vi "4Linea1.vi"(11 "array":string[][](array[string])) -> (3 "x .or. y?":bool)   [LabVIEW 2020]
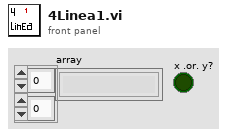
[diagram p1: front panel]
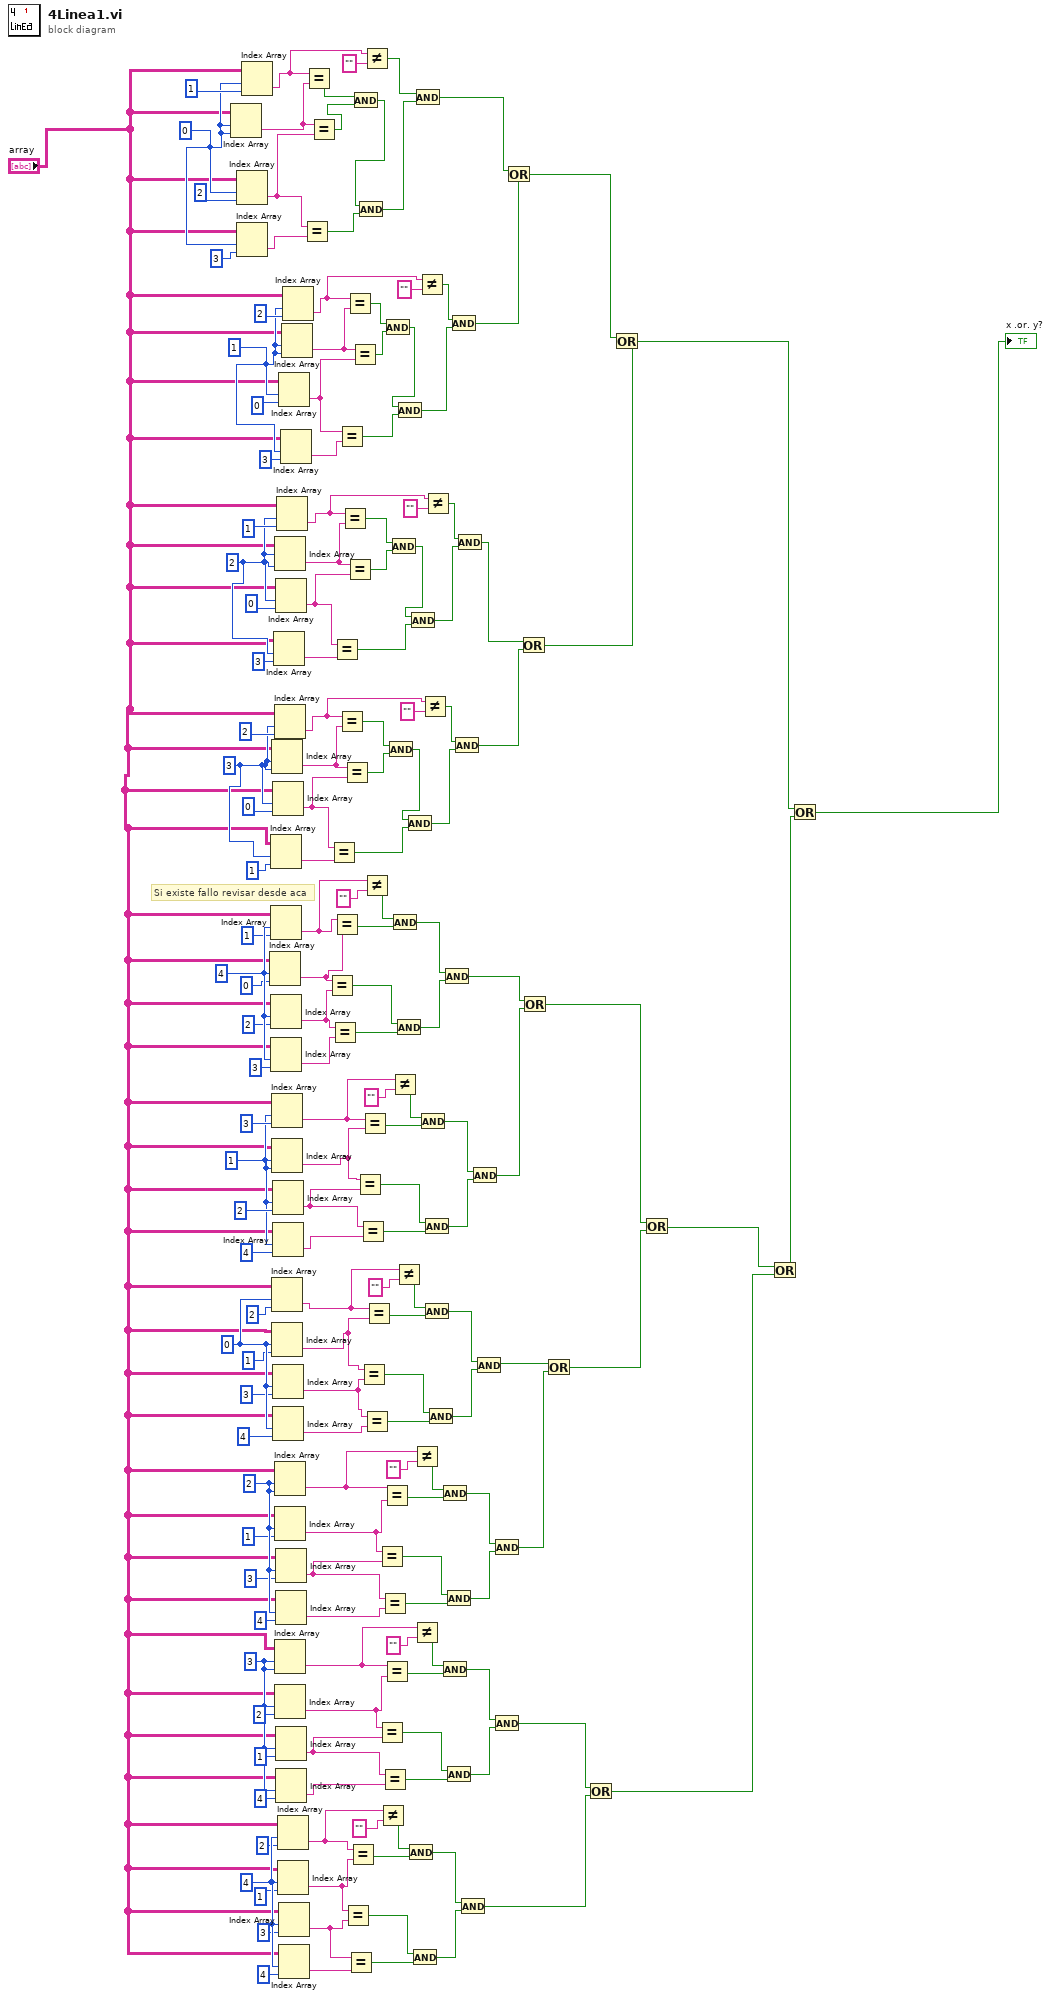
[diagram p0: block diagram]
diagram:
  w20 = 4 ("index (row)")
  w54 = 3 ("index (row)")
  w58 = 2 ("index (row)")
  w63 = 0 ("index (row)")
  w89 = 1 ("index (row)")
  w107 = 4 ("index (row)")
  w116 = 3
  w131 = 2
  w138 = 1
  w146 = 0
  # "Si existe fallo revisar desde aca"
  n1 = Index Array(array="array", index (row)=w146, index (col)=w146) -> (element=w171:string)
  n2 = Index Array(array="array", index (row)=w146, index (col)=2) -> (element=w144:string)
  n3 = Index Array(array="array", index (row)=w146, index (col)=3) -> (element=w143:string)
  n4 = Index Array(array="array", index (row)=w146, index (col)=1) -> (element=w152:string)
  n5 = Index Array(array="array", index (row)=w107, index (col)=0 ("disabled index (col)")) -> (element=w101:string)
  n6 = Index Array(array="array", index (row)=w116, index (col)=1) -> (element=w114:string)
  n7 = Index Array(array="array", index (row)=w107, index (col)=1 ("disabled index (col)")) -> (element=w102:string)
  n8 = Index Array(array="array", index (row)=w107, index (col)=2 ("disabled index (col)")) -> (element=w100:string)
  n9 = Index Array(array="array", index (row)=w107, index (col)=3 ("disabled index (col)")) -> (element=w99:string)
  n10 = Index Array(array="array", index (row)=w116, index (col)=w116) -> (element=w123:string)
  n11 = Index Array(array="array", index (row)=w89, index (col)=3 ("disabled index (col)")) -> (element=w80:string)
  n12 = Index Array(array="array", index (row)=w89, index (col)=w89) -> (element=w79:string)
  n13 = Index Array(array="array", index (row)=w63, index (col)=2 ("disabled index (col)")) -> (element=w69:string)
  n14 = Index Array(array="array", index (row)=w63, index (col)=1 ("disabled index (col)")) -> (element=w66:string)
  n15 = Index Array(array="array", index (row)=w116, index (col)=0) -> (element=w115:string)
  n16 = Index Array(array="array", index (row)=w89, index (col)=2 ("disabled index (col)")) -> (element=w78:string)
  n17 = Index Array(array="array", index (row)=w89, index (col)=4 ("disabled index (col)")) -> (element=w77:string)
  n18 = Index Array(array="array", index (row)=w63, index (col)=3 ("disabled index (col)")) -> (element=w68:string)
  n19 = Index Array(array="array", index (row)=w63, index (col)=4 ("disabled index (col)")) -> (element=w67:string)
  n20 = Index Array(array="array", index (row)=w131, index (col)=3) -> (element=w129:string)
  n21 = Index Array(array="array", index (row)=w131, index (col)=w131) -> (element=w165:string)
  n22 = Index Array(array="array", index (row)=w116, index (col)=2) -> (element=w119:string)
  n23 = Index Array(array="array", index (row)=w58, index (col)=w58) -> (element=w30:string)
  n24 = Index Array(array="array", index (row)=w58, index (col)=1 ("disabled index (col)")) -> (element=w29:string)
  n25 = Index Array(array="array", index (row)=w54, index (col)=w54) -> (element=w23:string)
  n26 = Index Array(array="array", index (row)=w54, index (col)=2) -> (element=w26:string)
  n27 = Index Array(array="array", index (row)=w131, index (col)=0) -> (element=w130:string)
  n28 = Index Array(array="array", index (row)=w58, index (col)=3 ("disabled index (col)")) -> (element=w28:string)
  n29 = Index Array(array="array", index (row)=w58, index (col)=4 ("disabled index (col)")) -> (element=w27:string)
  n30 = Index Array(array="array", index (row)=w54, index (col)=1) -> (element=w25:string)
  n31 = Index Array(array="array", index (row)=w54, index (col)=4) -> (element=w24:string)
  n32 = Index Array(array="array", index (row)=w131, index (col)=1) -> (element=w161:string)
  n33 = Index Array(array="array", index (row)=w20, index (col)=2) -> (element=w13:string)
  n34 = Index Array(array="array", index (row)=w20, index (col)=1) -> (element=w12:string)
  n35 = Index Array(array="array", index (row)=w138, index (col)=0) -> (element=w134:string)
  n36 = Index Array(array="array", index (row)=w20, index (col)=3) -> (element=w11:string)
  n37 = Index Array(array="array", index (row)=w20, index (col)=4) -> (element=w10:string)
  n38 = Index Array(array="array", index (row)=w138, index (col)=3) -> (element=w135:string)
  n39 = Index Array(array="array", index (row)=w138, index (col)=w138) -> (element=w168:string)
  n40 = Index Array(array="array", index (row)=w138, index (col)=2) -> (element=w155:string)
  n41 = Equal?(x=w144, y=w143) -> (x = y?=w142:bool)
  n42 = Equal?(x=w152, y=w171) -> (x = y?=w151:bool)
  n43 = Equal?(x=w171, y=w144) -> (x = y?=w150:bool)
  n44 = Equal?(x=w101, y=w100) -> (x = y?=w95:bool)
  n45 = Equal?(x=w115, y=w114) -> (x = y?=w113:bool)
  n46 = Equal?(x=w100, y=w99) -> (x = y?=w94:bool)
  n47 = Equal?(x=w130, y=w129) -> (x = y?=w128:bool)
  n48 = Equal?(x=w102, y=w101) -> (x = y?=w96:bool)
  n49 = Equal?(x=w134, y=w135) -> (x = y?=w137:bool)
  n50 = Equal?(x=w119, y=w123) -> (x = y?=w122:bool)
  n51 = Equal?(x=w161, y=w165) -> (x = y?=w164:bool)
  n52 = Equal?(x=w123, y=w115) -> (x = y?=w121:bool)
  n53 = Equal?(x=w12, y=w11) -> (x = y?=w34:bool)
  n54 = Equal?(x=w155, y=w168) -> (x = y?=w157:bool)
  n55 = Equal?(x=w165, y=w130) -> (x = y?=w163:bool)
  n56 = Equal?(x=w11, y=w10) -> (x = y?=w33:bool)
  n57 = Equal?(x=w13, y=w12) -> (x = y?=w35:bool)
  n58 = Equal?(x=w168, y=w134) -> (x = y?=w156:bool)
  n59 = And(x=w151, y=w150) -> (x .and. y?=w141:bool)
  n60 = Equal?(x=w79, y=w78) -> (x = y?=w84:bool)
  n61 = And(x=w141, y=w142) -> (x .and. y?=w140:bool)
  n62 = Equal?(x=w78, y=w77) -> (x = y?=w83:bool)
  n63 = Equal?(x=w66, y=w68) -> (x = y?=w73:bool)
  n64 = Equal?(x=w80, y=w79) -> (x = y?=w85:bool)
  n65 = Not Equal?(x=w152, y="") -> (x != y?=w153:bool)
  n66 = Not Equal?(x=w102, y="") -> (x != y?=w97:bool)
  n67 = Equal?(x=w68, y=w67) -> (x = y?=w72:bool)
  n68 = Equal?(x=w69, y=w66) -> (x = y?=w74:bool)
  n69 = Equal?(x=w29, y=w28) -> (x = y?=w47:bool)
  n70 = Equal?(x=w26, y=w25) -> (x = y?=w40:bool)
  n71 = Not Equal?(x=w13, y="") -> (x != y?=w36:bool)
  n72 = Equal?(x=w28, y=w27) -> (x = y?=w46:bool)
  n73 = Equal?(x=w25, y=w24) -> (x = y?=w39:bool)
  n74 = Equal?(x=w30, y=w29) -> (x = y?=w48:bool)
  n75 = Equal?(x=w23, y=w26) -> (x = y?=w41:bool)
  n76 = And(x=w157, y=w156) -> (x .and. y?=w136:bool)
  n77 = And(x=w122, y=w121) -> (x .and. y?=w112:bool)
  n78 = And(x=w164, y=w163) -> (x .and. y?=w127:bool)
  n79 = And(x=w97, y=w96) -> (x .and. y?=w93:bool)
  n80 = Not Equal?(x=w80, y="") -> (x != y?=w86:bool)
  n81 = And(x=w95, y=w94) -> (x .and. y?=w92:bool)
  n82 = Not Equal?(x=w69, y="") -> (x != y?=w75:bool)
  n83 = And(x=w136, y=w137) -> (x .and. y?=w133:bool)
  n84 = And(x=w112, y=w113) -> (x .and. y?=w111:bool)
  n85 = And(x=w36, y=w35) -> (x .and. y?=w32:bool)
  n86 = And(x=w127, y=w128) -> (x .and. y?=w126:bool)
  n87 = And(x=w34, y=w33) -> (x .and. y?=w31:bool)
  n88 = Not Equal?(x=w30, y="") -> (x != y?=w49:bool)
  n89 = Not Equal?(x=w23, y="") -> (x != y?=w42:bool)
  n90 = And(x=w153, y=w140) -> (x .and. y?=w149:bool)
  n91 = Not Equal?(x=w155, y="") -> (x != y?=w158:bool)
  n92 = And(x=w86, y=w85) -> (x .and. y?=w82:bool)
  n93 = Not Equal?(x=w119, y="") -> (x != y?=w118:bool)
  n94 = And(x=w84, y=w83) -> (x .and. y?=w81:bool)
  n95 = And(x=w75, y=w74) -> (x .and. y?=w71:bool)
  n96 = Not Equal?(x=w161, y="") -> (x != y?=w160:bool)
  n97 = And(x=w73, y=w72) -> (x .and. y?=w70:bool)
  n98 = And(x=w49, y=w48) -> (x .and. y?=w45:bool)
  n99 = And(x=w42, y=w41) -> (x .and. y?=w38:bool)
  n100 = And(x=w93, y=w92) -> (x .and. y?=w65:bool)
  n101 = And(x=w47, y=w46) -> (x .and. y?=w44:bool)
  n102 = And(x=w40, y=w39) -> (x .and. y?=w37:bool)
  n103 = And(x=w158, y=w133) -> (x .and. y?=w148:bool)
  n104 = And(x=w118, y=w111) -> (x .and. y?=w109:bool)
  n105 = And(x=w160, y=w126) -> (x .and. y?=w110:bool)
  n106 = And(x=w32, y=w31) -> (x .and. y?=w8:bool)
  n107 = And(x=w82, y=w81) -> (x .and. y?=w64:bool)
  n108 = And(x=w71, y=w70) -> (x .and. y?=w21:bool)
  n109 = And(x=w45, y=w44) -> (x .and. y?=w22:bool)
  n110 = And(x=w38, y=w37) -> (x .and. y?=w9:bool)
  n111 = Or(x=w149, y=w148) -> (x .or. y?=w147:bool)
  n112 = Or(x=w110, y=w109) -> (x .or. y?=w108:bool)
  n113 = Or(x=w65, y=w64) -> (x .or. y?=w7:bool)
  n114 = Or(x=w21, y=w22) -> (x .or. y?=w6:bool)
  n115 = Or(x=w9, y=w8) -> (x .or. y?=w5:bool)
  n116 = Or(x=w147, y=w108) -> (x .or. y?=w2:bool)
  n117 = Or(x=w7, y=w6) -> (x .or. y?=w4:bool)
  n118 = Or(x=w4, y=w5) -> (x .or. y?=w3:bool)
  n119 = Or(x=w2, y=w3) -> (x .or. y?=→"x .or. y?":bool)
